vi "Agilent 34401 Read Temperature Measurement (RTD).vi"() -> ()   [LabVIEW 2016]
doc: "This example shows how to configure a temperature measurement on an RTD probe and take a single reading.\n\n<B>Note:</B>\n\n(1) This example only applies to the Agilent 34410/34411 models."
uses:
  <vilib>/Utility/error.llb/DialogType.ctl
  <instrlib>/Agilent 34401/Public/Configure/Configure Temperature (RTD).vi
  <instrlib>/Agilent 34401/Public/Data/Read (Single Point).vi
  <instrlib>/Agilent 34401/Agilent 34401.lvlib
panel:
  in  "Unit (0: Celsius)":u16(ring) items=["C", "F", "K"]
  in  "Wire Mode (1: 4-Wire)":i16(ring)=1 items=["2-Wire", "4-Wire"]
  in  "Enable Offset Compensation (F: Disable)":bool
  in  "VISA resource name":refnum<visa-resource-name>
  out "Measurement":dbl
  in  "Nominal Resistance (100 ohms)":dbl=100.0
  # "(c) 2005-2015 National Instruments.  ALL RIGHTS RESERVED."
  # "Note: This example only applies to the 34410A/34411A models."
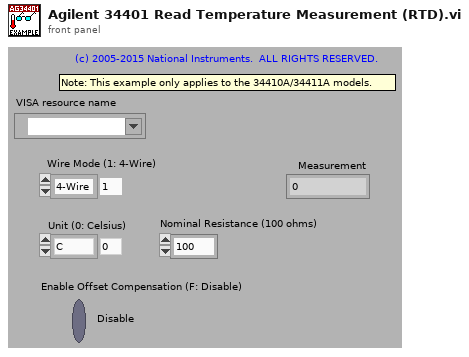
[diagram p1: front panel]
types:
  T1 = typedef "DialogType.ctl" = u16
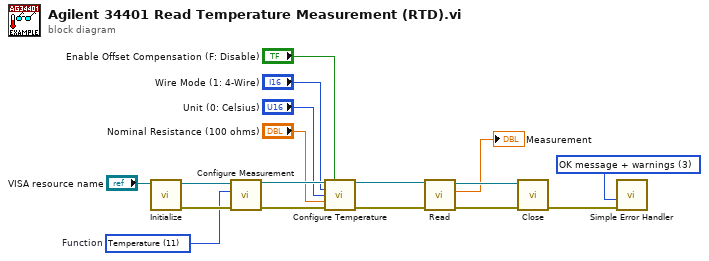
[diagram p0: block diagram]
diagram:
  w3 = T1 3 items=["no dialog", "OK message", "continue or stop message", "OK message + warnings", "continue/stop + warnings"] ("type of dialog (OK msg:1)")
  w8 = u16 11 items=["DC Voltage", "AC Voltage", "2 - Wire Resistance", "4 - Wire Resistance", "DC Current", "AC Current", "Frequency", "Period", "Continuity", "Diode Checking", "VDC:VDC Ratio", "Temperature", "Capacitance"]  # Function
  n1 = call <instrlib>:"Initialize.vi"("VISA resource name"="VISA resource name") -> ("error out"=w17:errorcluster, "VISA resource name out"=w16:refnum<visa-resource-name>)  [unwired: 9 in]
  n2 = call <instrlib>:"Configure Measurement.vi"("error in (no error)"=w17, "Function (0: DC Voltage)"=w8, "VISA resource name"=w16) -> ("error out"=w15:errorcluster, "VISA resource name out"=w14:refnum<visa-resource-name>)  [unwired: 7 in]
  n3 = call-poly <instrlib>:"Configure Temperature.vi"("VISA resource name"=w14, "Enable Offset Compensation (F: Disable)"="Enable Offset Compensation (F: Disable)", "Wire Mode (1: 4-Wire)"="Wire Mode (1: 4-Wire)", "Unit (0: Celsius)"="Unit (0: Celsius)", "Nominal Resistance (100 ohms)"="Nominal Resistance (100 ohms)", "error in (no error)"=w15) -> ("VISA resource name out"=w12:refnum<visa-resource-name>, "error out"=w13:errorcluster)  [unwired: 8 in]
  n4 = call-poly <instrlib>:"Read.vi"("error in (no error)"=w13, "VISA resource name"=w12) -> ("error out"=w11:errorcluster, "Measurement"=→"Measurement":dbl, "VISA resource name out"=w10:refnum<visa-resource-name>)  [unwired: 7 in]
  n5 = call <instrlib>:"Close.vi"("error in (no error)"=w11, "VISA resource name"=w10) -> ("error out"=w9:errorcluster)  [unwired: 9 in]
  n6 = call <vilib>:"Simple Error Handler.vi"("type of dialog (OK msg:1)"=w3, "error in (no error)"=w9) -> ()  [unwired: 3 in, 5 out]
